vi "Loadcell Control Motor.vi"() -> ()   [LabVIEW 2020]
panel:
  in  "Motor Trottle":dbl(slide) scale=0.0..5.0
  out "Round":dynamicdata(graph)
  out "data":dynamicdata(graph)
  in  "stop (F)":bool
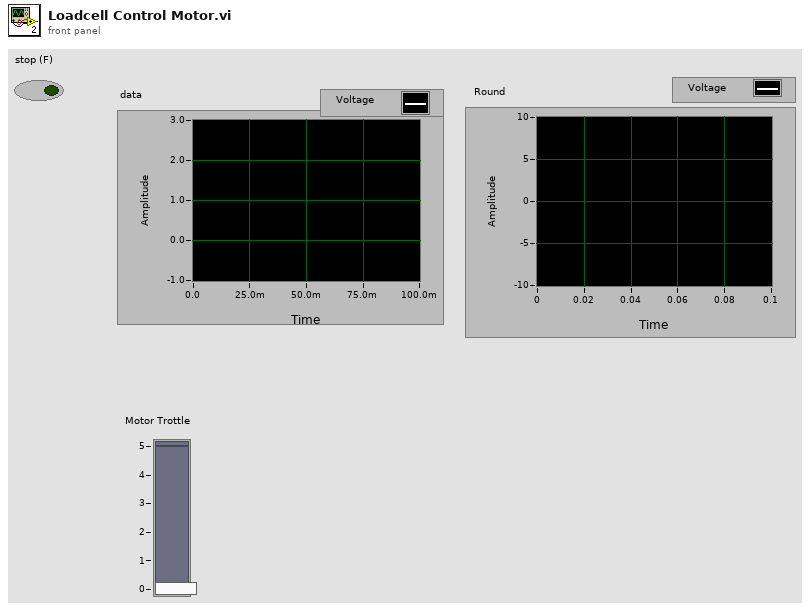
[diagram p1: front panel]
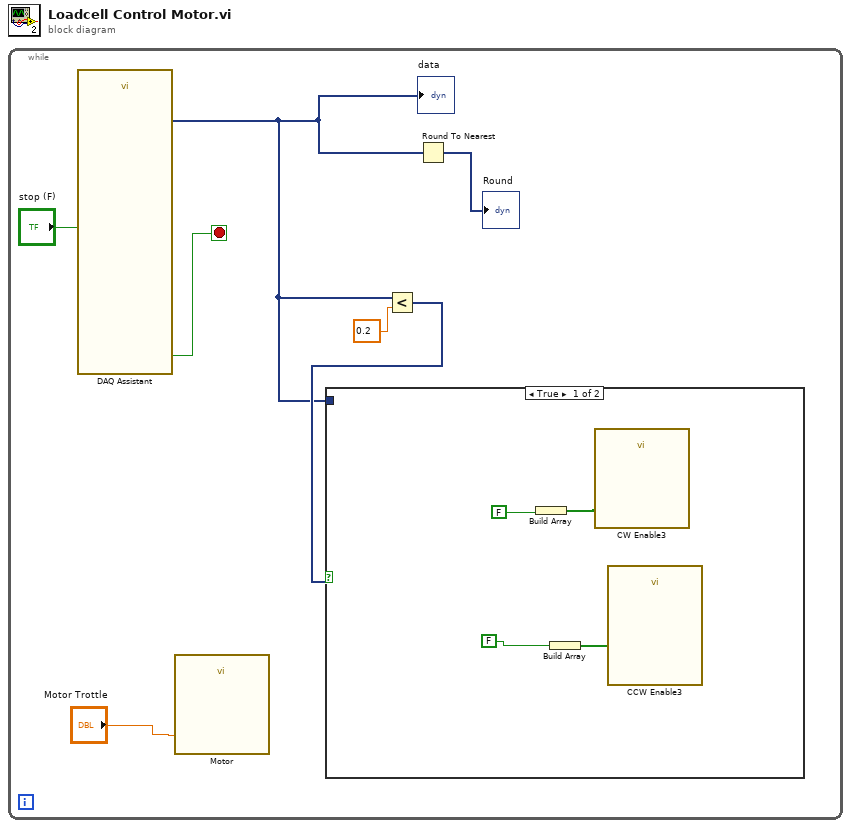
[diagram p0: block diagram]
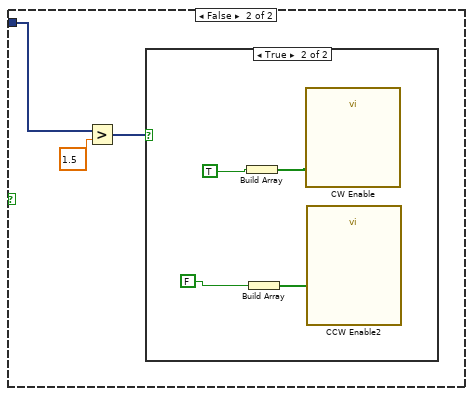
[diagram p2: hidden frame]
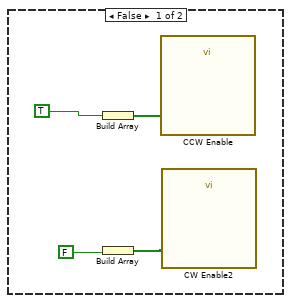
[diagram p3: hidden frame]
diagram:
  n1 = while {
    stop <- w5 stop-if-true
    n2 = call "DAQ Assistant"("stop (F)"="stop (F)") -> ("data"=w1:dynamicdata, "stopped"=w5:bool)  [unwired: 15 in, 2 out]
    "data" <- w1
    n3 = call "Motor"("data"="Motor Trottle") -> ()  [unwired: 17 in, 2 out]
    n4 = Less?(x=w1, y=0.2) -> (x < y?=w2:dynamicdata)
    n5 = case shown="True" w2 {
      tunnel: w1 -> [_ w12]
      frame True {
        n6 = Build Array(FALSE) -> (w11:bool[])
        n7 = Build Array(FALSE) -> (w9:bool[])
        n8 = call "CW Enable3"("data"=w11) -> ()  [unwired: 17 in, 2 out]
        n9 = call "CCW Enable3"("data"=w9) -> ()  [unwired: 17 in, 2 out]
      }
      frame False {
        n10 = Greater?(x=w12, y=1.5) -> (0:w13:dynamicdata)
        n11 = case shown="True" w13 {
          frame False {
            n12 = Build Array(TRUE) -> (w18:bool[])
            n13 = Build Array(FALSE) -> (w16:bool[])
            n14 = call "CCW Enable"("data"=w18) -> ()  [unwired: 17 in, 2 out]
            n15 = call "CW Enable2"("data"=w16) -> ()  [unwired: 17 in, 2 out]
          }
          frame True {
            n16 = Build Array "Build Array"(TRUE) -> (w21:bool[])
            n17 = Build Array(FALSE) -> (w20:bool[])
            n18 = call "CW Enable"("data"=w21) -> ()  [unwired: 17 in, 2 out]
            n19 = call "CCW Enable2"("data"=w20) -> ()  [unwired: 17 in, 2 out]
          }
        }
      }
    }
    n20 = Round To Nearest(number=w1) -> (nearest integer value=→"Round":dynamicdata)
  }
